vi "Analysis.Count Occurrances, Funct Global, Str.vi"(10 "Item In":string, 11 "Reset":bool) -> (2 "Count List":i32[](array[numeric]), 3 "Item List":string[](array[string]), 5 "Added":bool)   [LabVIEW 2024]
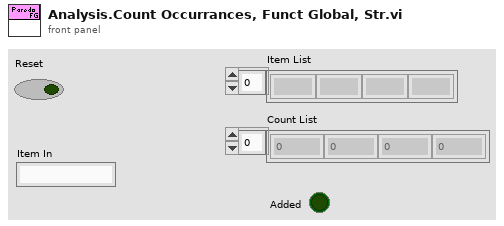
[diagram p1: front panel]
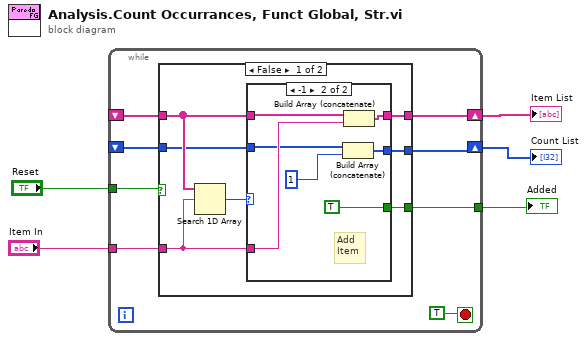
[diagram p0: block diagram]
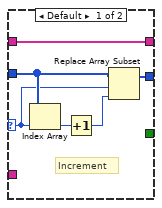
[diagram p2: hidden frame]
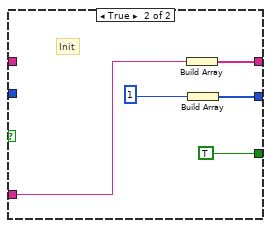
[diagram p3: hidden frame]
diagram:
  n1 = while {
    tunnel: "Item In" -> [w13]
    tunnel: [w10] -> w3
    shift-right: [w12] -> w4
    shift-left: _ -> [w11]
    tunnel: "Reset" -> [w8]
    shift-right: [w6] -> w1
    shift-left: _ -> [w7]
    stop <- TRUE stop-if-true
    n2 = case shown="False" w8 {
      tunnel: w13 -> [w20 w37]
      tunnel: [w19 w38] -> w12
      tunnel: w11 -> [w18 _]
      tunnel: [w16 TRUE] -> w10
      tunnel: w7 -> [w15 _]
      tunnel: [w14 w35] -> w6
      frame False {
        n3 = Search 1D Array(1D array=w18, element=w20) -> (index of element=w17:i32)  [unwired: 1 in]
        n4 = case shown="-1" w17 {
          selector: w17 -> [w23 _]
          tunnel: w20 -> [_ w31]
          tunnel: w18 -> [w26 w33]
          tunnel: [w26 w32] -> w19
          tunnel: [_ TRUE] -> w16
          tunnel: w15 -> [w24 w29]
          tunnel: [w25 w27] -> w14
          frame Default {
            # "Increment"
            n5 = Index Array(array=w24, index=w23) -> (element=w22:i32)
            n6 = Increment(x=w22) -> (x+1=w21:i32)
            n7 = Replace Array Subset(array=w24, new element=w21, index=w23) -> (w25:i32[])
          }
          frame -1 {
            # "Add\nItem"
            n8 = Build Array (concatenate)(w29, 1) -> (w27:i32[])
            n9 = Build Array (concatenate)(w33, w31) -> (w32:string[])
          }
        }
      }
      frame True {
        # "Init"
        n10 = Build Array(w37) -> (w38:string[])
        n11 = Build Array(1) -> (w35:i32[])
      }
    }
  }
  "Item List" <- w4
  "Added" <- w3
  "Count List" <- w1
